vi "FPGA_InterruptReadConfiguration.vi"(8 "error in (no error)":errorcluster, 11 "InteruptRef in":T5) -> (0 "error out":errorcluster, 1 "RisingEdge":bool, 2 "Source":T1={"DevStatus"={"status"=FALSE, "code"=0, "source"=""}, "AnalogTriggerMode?"=FALSE, "DigitalMode"={"DIO Channel"=enum."DIO 1"}, "AnalogTriggerMode"={"AnalogTriggerIndex"=enum."Trig 0", "OutputType"=enum."InWindow"}}, 3 "InteruptRef out":T5, 4 "FallingEdge":bool, 5 "WaitForAck":bool)   [LabVIEW 2017]
uses:
  <vilib>/Rock Robotics/SystemInterfaces/Interrupt/FPGA_InterruptRef.ctl
  <vilib>/Rock Robotics/SystemInterfaces/Interrupt/FPGA_InterruptIndex.ctl
  <vilib>/Rock Robotics/SystemInterfaces/CounterEncoderSourceConvertion/FPGA_CounterEncoderSourceConvertionLVSourceType.ctl
  <vilib>/Rock Robotics/SystemInterfaces/DIO/FPGA_DIODigitalSourceChannel.ctl
  <vilib>/Rock Robotics/SystemInterfaces/AnalogTrigger/FPGA_AnalogTriggerIndex.ctl
  <vilib>/Rock Robotics/SystemInterfaces/AnalogTrigger/FPGA_AnalogTriggerOutType.ctl
  <vilib>/Rock Robotics/SystemInterfaces/System/FPGA_SystemFPGA Ref Global.vi
  <vilib>/Utility/error.llb/Error Cluster From Error Code.vi
  <vilib>/rvi/errors/niLvFpgaAdjustHostInterfaceError.vi
  <vilib>/rvi/interface/nirviReadWriteControl/nirviReadWriteControl.xnode
  <vilib>/Rock Robotics/SystemInterfaces/System/FPGA_SystemFRC FPGA Ref.ctl
  NiFpgaLv.dll
  <vilib>/rvi/interface/Simulation/niFpgaSimulationCallBeginRW.vi
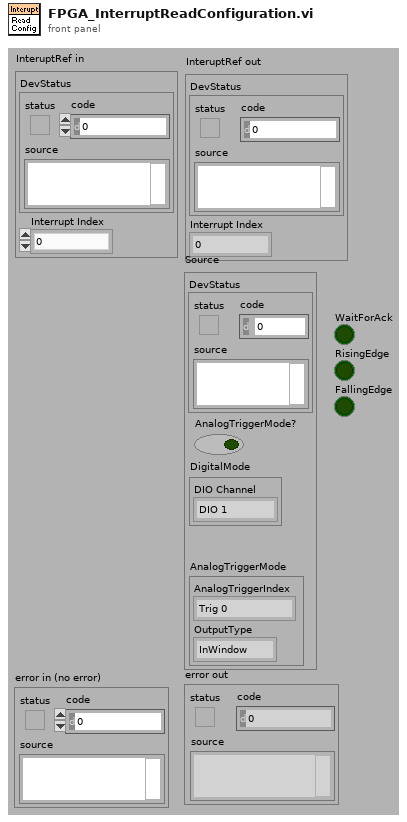
[diagram p1: front panel]
types:
  T1 = typedef "FPGA_CounterEncoderSourceConvertionLVSourceType.ctl" = cluster{"DevStatus":errorcluster, "AnalogTriggerMode?":bool, "DigitalMode":cluster{"DIO Channel":T2}, "AnalogTriggerMode":cluster{"AnalogTriggerIndex":T3, "OutputType":T4}}
  T2 = typedef "FPGA_DIODigitalSourceChannel.ctl" = enum8{"DIO 0", "DIO 1", "DIO 2", "DIO 3", "DIO 4", "DIO 5", "DIO 6", "DIO 7", "DIO 8", "DIO 9", "DIO MXP 0", "DIO MXP 1", "DIO MXP 2", "DIO MXP 3", "DIO MXP 4", "DIO MXP 5", "DIO MXP 6", "DIO MXP 7", "DIO MXP 8", "DIO MXP 9", "DIO MXP 10", "DIO MXP 11", "DIO MXP 12", "DIO MXP 13", "DIO MXP 14", "DIO MXP 15", "Disabled"}
  T3 = typedef "FPGA_AnalogTriggerIndex.ctl" = enum8{"Trig 0", "Trig 1", "Trig 2", "Trig 3", "Trig 4", "Trig 5", "Trig 6", "Trig 7", "Invalid"}
  T4 = typedef "FPGA_AnalogTriggerOutType.ctl" = enum16{"InWindow", "TriggerState", "Rising", "Falling"}
  T5 = typedef "FPGA_InterruptRef.ctl" = cluster{"DevStatus":errorcluster, "Interrupt Index":T6}
  T6 = typedef "FPGA_InterruptIndex.ctl" = enum8{"0", "1", "2", "3", "4", "5", "6", "7", "Invalid"}
  T7 = typedef "FPGA_SystemFRC FPGA Ref.ctl" = refnum<k20>
  T8 = cluster{"Source":cluster{"Channel":fxp<+,4,4>, "Module":fxp<+,1,1>, "AnalogTrigger":bool}, "RisingEdge":bool, "FallingEdge":bool, "WaitForAck":bool}
  T9 = cluster{"Channel":fxp<+,4,4>, "Module":fxp<+,1,1>, "AnalogTrigger":bool}
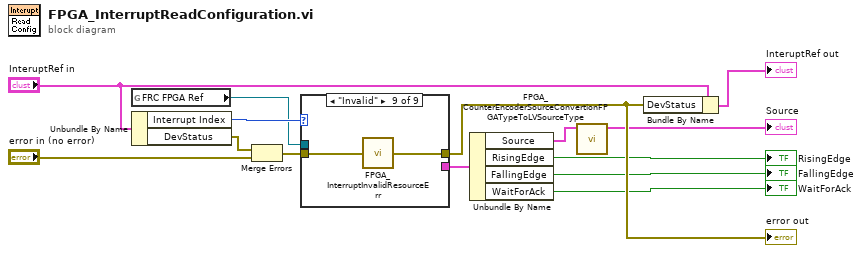
[diagram p0: block diagram]
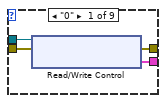
[diagram p2: hidden frame]
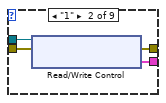
[diagram p3: hidden frame]
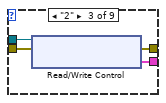
[diagram p4: hidden frame]
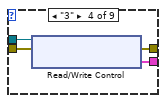
[diagram p5: hidden frame]
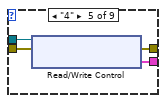
[diagram p6: hidden frame]
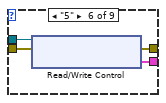
[diagram p7: hidden frame]
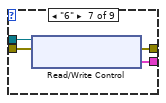
[diagram p8: hidden frame]
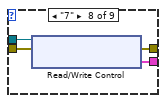
[diagram p9: hidden frame]
diagram:
  n1 = global read "FPGA_SystemFPGA Ref Global.vi" "FRC FPGA Ref"() -> (w3:T7)
  n2 = Unbundle By Name("InteruptRef in") -> ("Interrupt Index"=w6:T6, "DevStatus"=w1:errorcluster)
  n3 = Merge Errors(w1, "error in (no error)") -> (w2:errorcluster)
  n4 = case shown="\"Invalid\"" w6 {
    tunnel: w3 -> [w17 w22 w26 w30 w34 w38 w42 w46 _]
    tunnel: w2 -> [w18 w21 w25 w29 w33 w37 w41 w45 w47]
    tunnel: [w16 w20 w24 w28 w32 w36 w40 w44 w48] -> w11
    tunnel: [w15 w19 w23 w27 w31 w35 w39 w43 _] -> w4
    frame "0" {
      n5 = xnode "Read/Write Control"("FPGA VI Reference In"=w17, "error in"=w18) -> ("error out"=w16:errorcluster, "Interrupt0.Config"=w15:T8)  [unwired: 1 out]
    }
    frame "1" {
      n6 = xnode "Read/Write Control"("FPGA VI Reference In"=w22, "error in"=w21) -> ("error out"=w20:errorcluster, "Interrupt1.Config"=w19:T8)  [unwired: 1 out]
    }
    frame "2" {
      n7 = xnode "Read/Write Control"("FPGA VI Reference In"=w26, "error in"=w25) -> ("error out"=w24:errorcluster, "Interrupt2.Config"=w23:T8)  [unwired: 1 out]
    }
    frame "3" {
      n8 = xnode "Read/Write Control"("FPGA VI Reference In"=w30, "error in"=w29) -> ("error out"=w28:errorcluster, "Interrupt3.Config"=w27:T8)  [unwired: 1 out]
    }
    frame "4" {
      n9 = xnode "Read/Write Control"("FPGA VI Reference In"=w34, "error in"=w33) -> ("error out"=w32:errorcluster, "Interrupt4.Config"=w31:T8)  [unwired: 1 out]
    }
    frame "5" {
      n10 = xnode "Read/Write Control"("FPGA VI Reference In"=w38, "error in"=w37) -> ("error out"=w36:errorcluster, "Interrupt5.Config"=w35:T8)  [unwired: 1 out]
    }
    frame "6" {
      n11 = xnode "Read/Write Control"("FPGA VI Reference In"=w42, "error in"=w41) -> ("error out"=w40:errorcluster, "Interrupt6.Config"=w39:T8)  [unwired: 1 out]
    }
    frame "7" {
      n12 = xnode "Read/Write Control"("FPGA VI Reference In"=w46, "error in"=w45) -> ("error out"=w44:errorcluster, "Interrupt7.Config"=w43:T8)  [unwired: 1 out]
    }
    frame "Invalid" {
      n13 = call <vilib>:"FPGA_InterruptInvalidResourceErr.vi"("error in (no error)"=w47) -> ("error out"=w48:errorcluster)
    }
  }
  "error out" <- w11
  n14 = Unbundle By Name(w4) -> ("Source"=w5:T9, "RisingEdge"=→"RisingEdge":bool, "FallingEdge"=→"FallingEdge":bool, "WaitForAck"=→"WaitForAck":bool)
  n15 = call <vilib>:"FPGA_CounterEncoderSourceConvertionFPGATypeToLVSourceType.vi"("FPGASource"=w5) -> ("DigitalSource"=→"Source":T1)  [unwired: 10 out]
  n16 = Bundle By Name(cluster="InteruptRef in", "DevStatus"=w11) -> (→"InteruptRef out":T5)
